vi "PWM Read Duty.vi"(7 "GPIO #":T1=-1, 8 "error in (no error)":errorcluster, 11 "VisaComms in":refnum<class "VisaComms.lvclass">) -> (0 "error out":errorcluster, 2 "Duty % (0-1)":sgl, 3 "VisaComms out":refnum<class "VisaComms.lvclass">)   [LabVIEW 2024, in "CTI.lvlib" / "VisaComms.lvclass"]
uses:
  VisaComms.lvclass
  GPIO Number.ctl
  VisaComms.lvclass/VisaComms.ctl
  Clean Visa Errors.vi
  CTI.lvlib
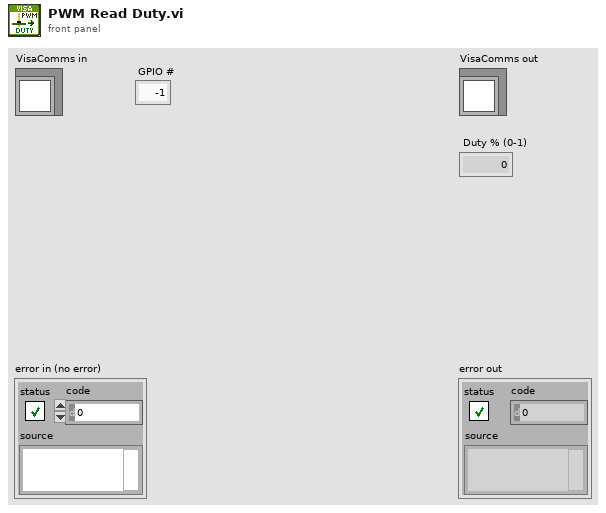
[diagram p1: front panel]
types:
  T1 = typedef "CTI.lvlib/GPIO Number.ctl" = i8
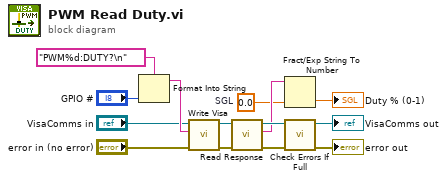
[diagram p0: block diagram]
diagram:
  w2 = sgl 0.0  # SGL
  n1 = Format Into String(format string="PWM%d:DUTY?\n", "GPIO #") -> (resulting string=w13:string)  [unwired: 2 in, 1 out]
  n2 = call "Write Visa.vi"("error in (no error)"="error in (no error)", "write buffer"=w13, "VisaComms in"="VisaComms in") -> ("error out"=w12:errorcluster, "VisaComms out"=w10:refnum<class "VisaComms.lvclass">)  [unwired: 6 in, 1 out]
  n3 = call "Read Response.vi"("error in (no error)"=w12, "VisaComms in"=w10) -> ("error out"=w11:errorcluster, "Response"=w4:string, "VisaComms out"=w9:refnum<class "VisaComms.lvclass">)  [unwired: 6 in, 1 out]
  n4 = Fract/Exp String To Number(string=w4, default (0 dbl)=w2) -> (number=→"Duty % (0-1)":sgl)  [unwired: 2 in, 1 out]
  n5 = call "Check Errors If Full.vi"("error in (no error)"=w11, "VisaComms in"=w9) -> ("error out"=→"error out":errorcluster, "VisaComms out"=→"VisaComms out":refnum<class "VisaComms.lvclass">)  [unwired: 8 in]
